vi "RandomData.vi"   [LabVIEW 2019]
uses:
  <vilib>/numeric/Random Number (Range) DBL.vi
types:
  T1 = enum16{"open", "replace", "create", "open or create", "replace or create", "replace or create with confirmation"}
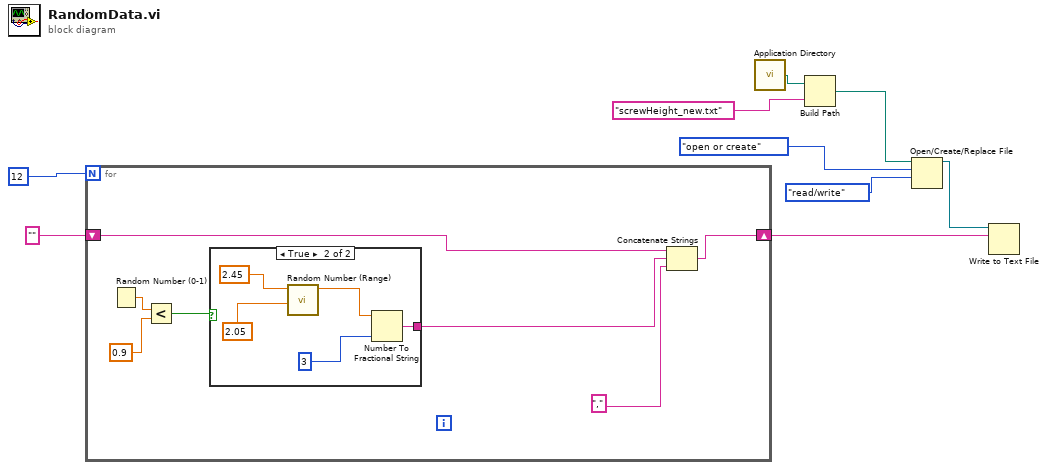
[diagram p0: block diagram]
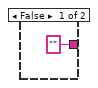
[diagram p2: hidden frame]
diagram:
  n1 = for {
    N: 12 -> [_]
    shift-right: [w15] -> w5
    shift-left: "" -> [w14]
    n2 = Random Number (0-1)() -> (number: 0 to 1=w13:dbl)
    n3 = Less?(x=w13, y=0.9) -> (x < y?=w11:bool)
    n4 = case shown="True" w11 {
      tunnel: ["" w18] -> w16
      frame False {
      }
      frame True {
        n5 = call-poly <vilib>:"Random Number (Range).vi"("lower bound (0)"=2.05, "upper bound (100)"=2.45) -> ("number"=w20:dbl)  [unwired: 9 in]
        n6 = Number To Fractional String(number=w20, precision (6)=i16 3) -> (F-format string=w18:string)  [unwired: 2 in]
      }
    }
    n7 = Concatenate Strings(w14, w16, "," ("string")) -> (w15:string)
  }
  n8 = call <vilib>:"Application Directory.vi"() -> ("Application Directory"=w7:path)
  n9 = Build Path(base path=w7, name or relative path="screwHeight_new.txt") -> (appended path=w4:path)
  n10 = Open/Create/Replace File(file path (use dialog)=w4, operation (0:open)=T1."open or create", access (0:read/write)=enum16{"read/write", "read-only", "write-only"}."read/write") -> (refnum out=w1:refnum<file>)  [unwired: 3 in, 2 out]
  n11 = Write to Text File(file (use dialog)=w1, text=w5) -> ()  [unwired: 2 in, 3 out]
